vi "dfd_Factor Decomposition.vi"(11 "number":i32) -> (1 "counts":i32[](array[numeric]), 2 "different factors":i32[](array[numeric]), 3 "factors":i32[](array[numeric]))   [LabVIEW 2017, in "NI_DigFilterLicensed.lvlib"]
uses:
  <vilib>/addons/Digital Filter Design/NI_DigFilterLicensed.lvlib
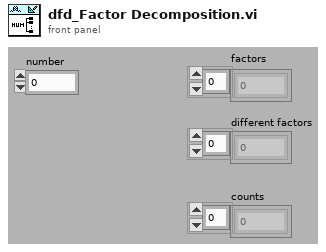
[diagram p1: front panel]
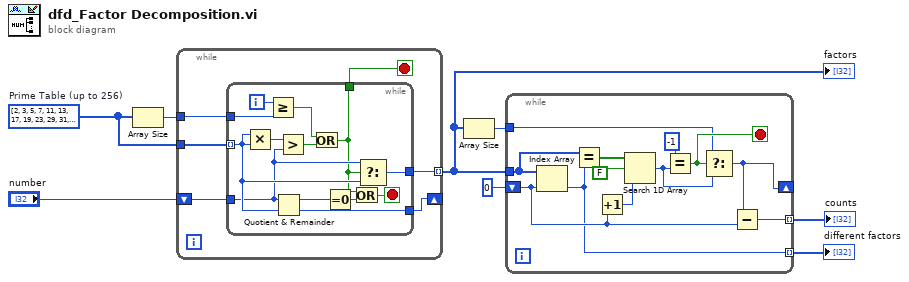
[diagram p0: block diagram]
diagram:
  w1 = i32[] [2, 3, 5, 7, 11, 13, 17, 19, 23, 29, 31, 37, 41, 43, 47, 53, 59, 61, 67, 71, 73, 79, 83, 89, 97, 101, 103, 107, 109, 113, 127, 131, 137, 139, 149, 151, 157, 163, 167, 173, 179, 181, 191, 193, 197, 199, 211, 223, 227, 229, 233, 239, 241, 251]  # Prime Table (up to 256)
  n1 = Array Size(array=w1) -> (size(s)=w8:i32)
  n2 = while {
    tunnel: [w11] -> w2 mode=indexing
    shift-left: "number" -> [w12]
    shift-right: [w9] -> _
    tunnel: w8 -> [w13]
    tunnel: w1 -> [w14]
    stop <- w10 stop-if-true
    n3 = while {
      tunnel: [w19] -> w10
      tunnel: [w25] -> w11
      tunnel: [w26] -> w9
      tunnel: w12 -> [w22]
      tunnel: w13 -> [w17]
      tunnel: w14 -> [w24] mode=indexing
      i -> [w18]
      stop <- w20 stop-if-true
      n4 = Multiply(x=w24, y=w24) -> (x*y=w23:i32)
      n5 = Greater Or Equal?(x=w18, y=w17) -> (x >= y?=w15:bool)
      n6 = Quotient & Remainder(x=w22, y=w24) -> (x-y*floor(x/y)=w27:i32, floor(x/y)=w26:i32)
      n7 = Greater?(x=w23, y=w22) -> (0:w16:bool)
      n8 = Or(x=w15, y=w16) -> (x .or. y?=w19:bool)
      n9 = Equal To 0?(x=w27) -> (x = 0?=w21:bool)
      n10 = Or(x=w19, y=w21) -> (x .or. y?=w20:bool)
      n11 = Select(t=w22, s=w19, f=w24) -> (s? t:f=w25:i32)
    }
  }
  "factors" <- w2
  n12 = Array Size(array=w2) -> (size(s)=w5:i32)
  n13 = while {
    tunnel: [w28] -> w4 mode=indexing
    tunnel: [w29] -> w3 mode=indexing
    tunnel: w5 -> [w32]
    shift-left: 0 -> [w30]
    shift-right: [w31] -> _
    tunnel: w2 -> [w39]
    stop <- w35 stop-if-true
    n14 = Index Array(array=w39, index=w30) -> (element=w28:i32)
    n15 = Equal?(x=w39, y=w28) -> (x = y?=w38:bool[])
    n16 = Increment(x=w30) -> (x+1=w36:i32)
    n17 = Search 1D Array(1D array=w38, element=FALSE, start index (0)=w36) -> (index of element=w33:i32)
    n18 = Equal?(x=-1 ("y"), y=w33) -> (x = y?=w35:bool)
    n19 = Select(t=w32, s=w35, f=w33) -> (s? t:f=w31:i32)
    n20 = Subtract(x=w31, y=w30) -> (x-y=w29:i32)
  }
  "different factors" <- w4
  "counts" <- w3
